vi "auto_irsuccess.vi"(9 "Direction":dbl, 10 "Skip IR":bool) -> (3 "Success":bool)   [LabVIEW 2010, in "LASA Beta.lvrbt"]
uses:
  LASA Beta.lvrbt
  op-run.vi
  op-read.vi
panel:
  # "Output"
  # "Skip IR beacon mode and just place if TRUE"
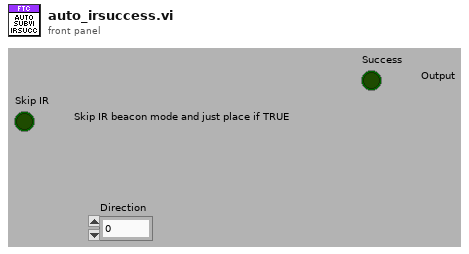
[diagram p1: front panel]
types:
  T1 = enum16{"Initialize", "Drive", "Math", "Move Back", "Exit"}
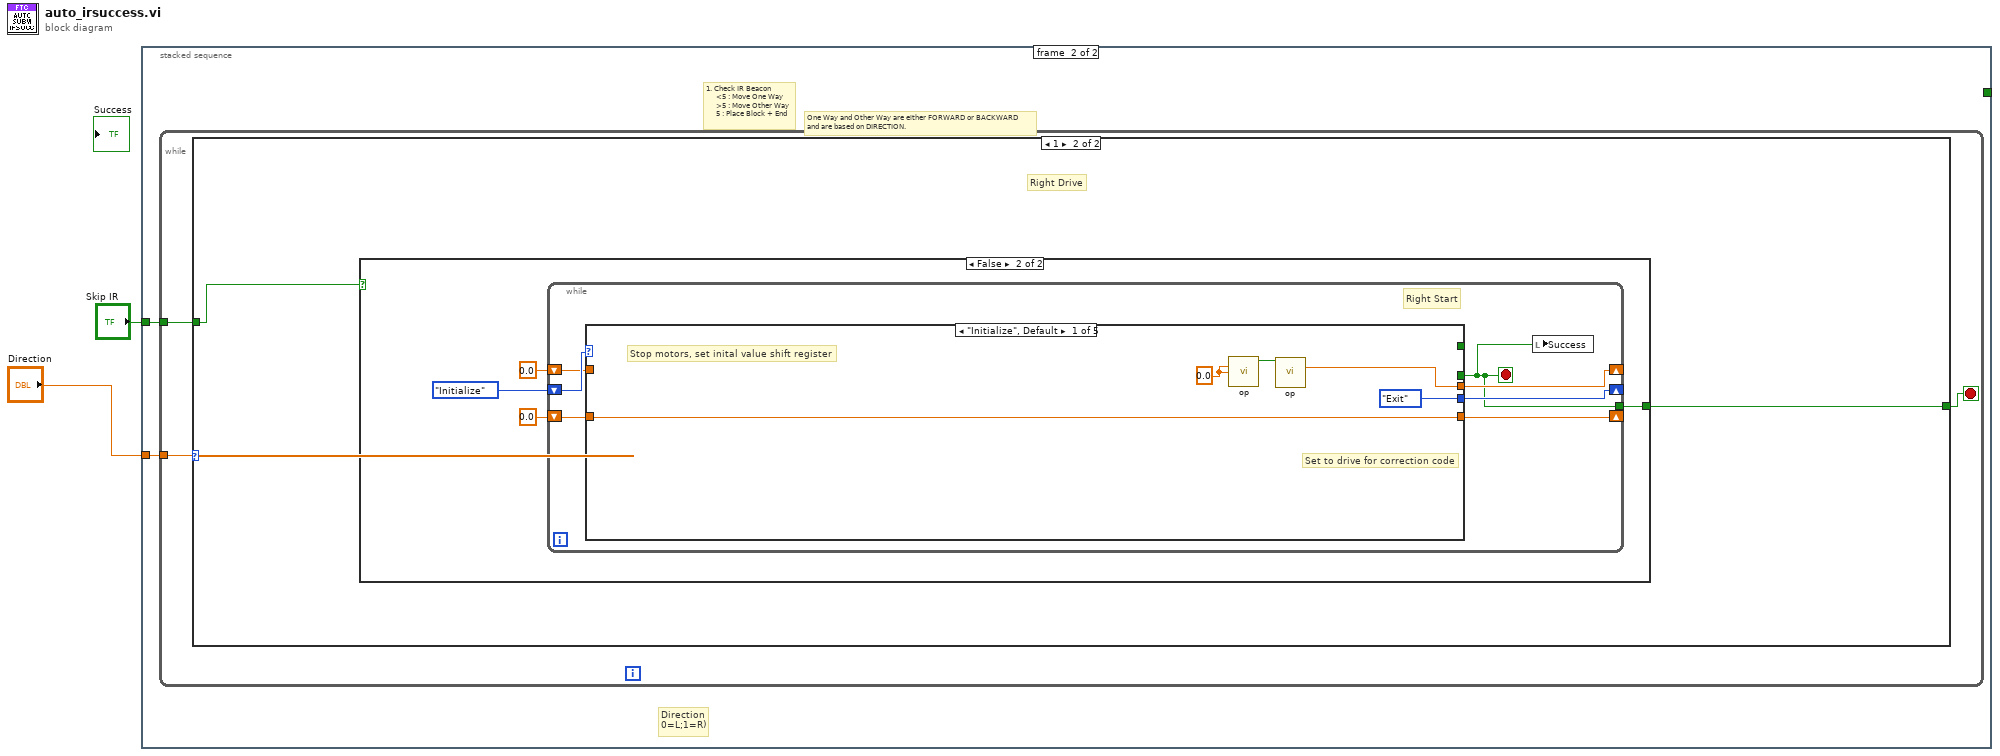
[diagram p0: block diagram]
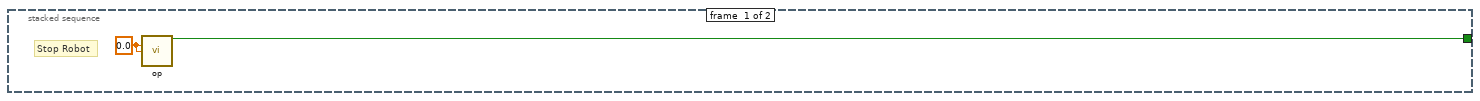
[diagram p2: hidden frame]
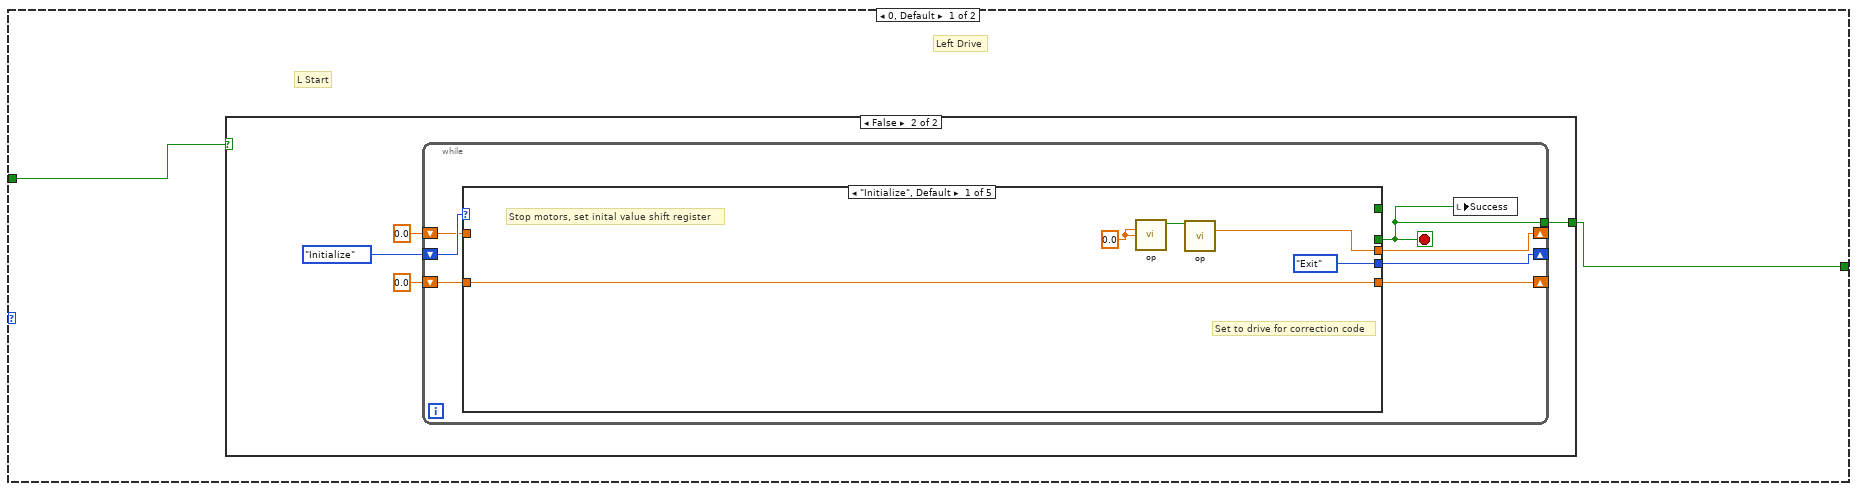
[diagram p3: hidden frame]
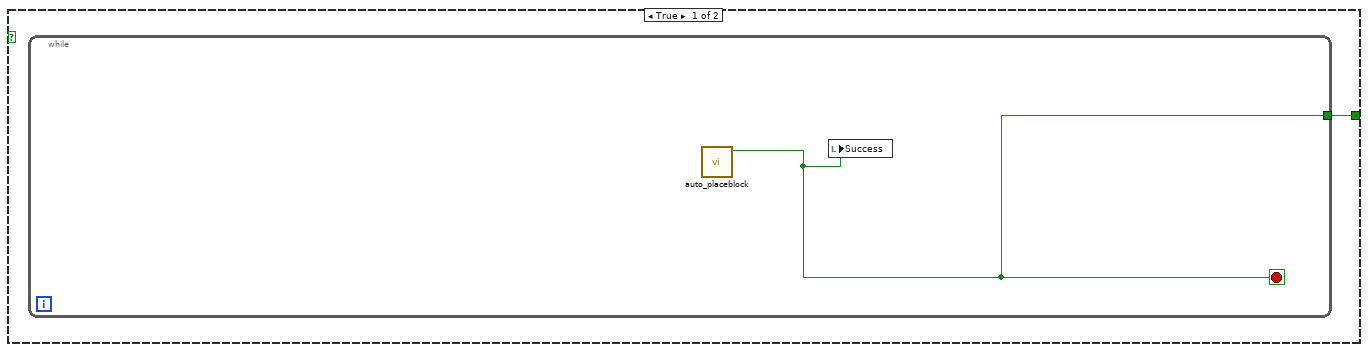
[diagram p4: hidden frame]
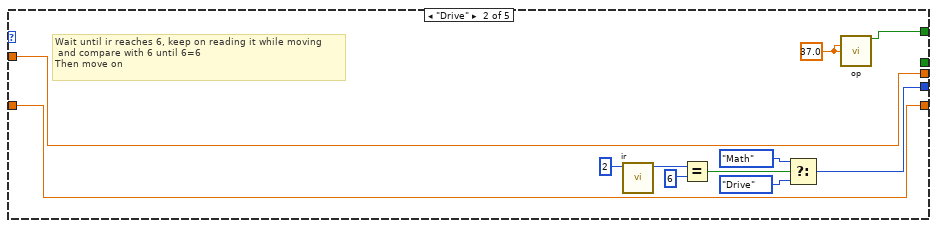
[diagram p5: hidden frame]
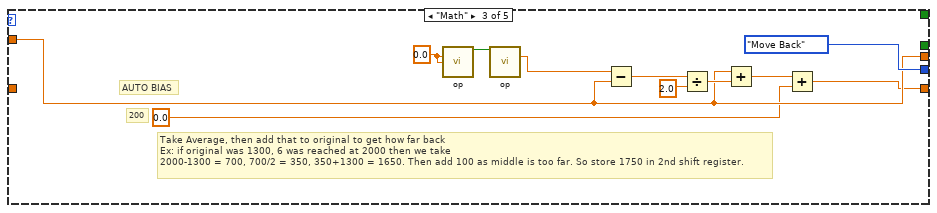
[diagram p6: hidden frame]
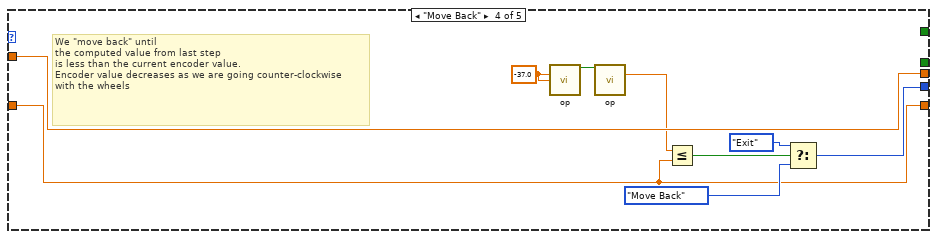
[diagram p7: hidden frame]
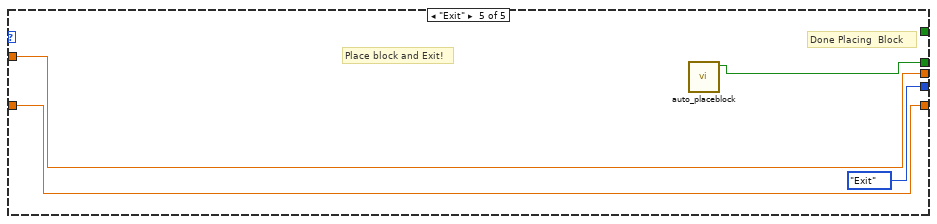
[diagram p8: hidden frame]
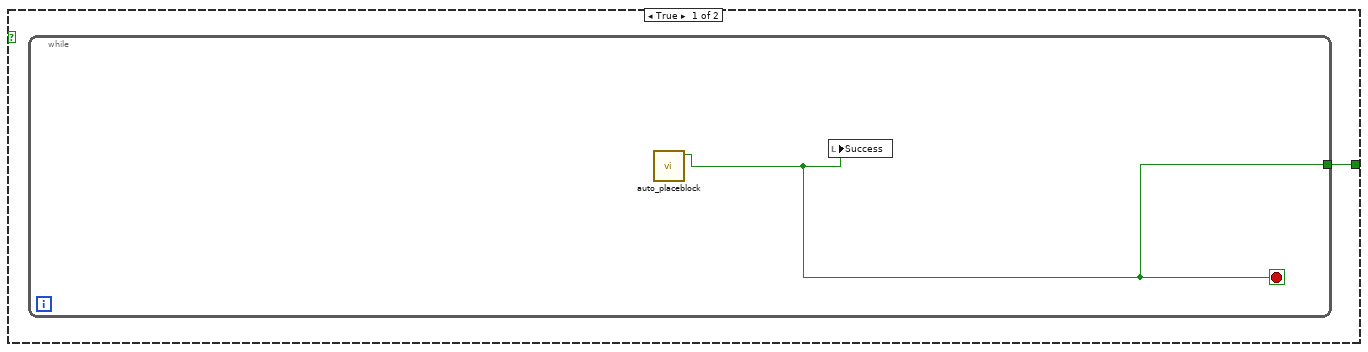
[diagram p9: hidden frame]
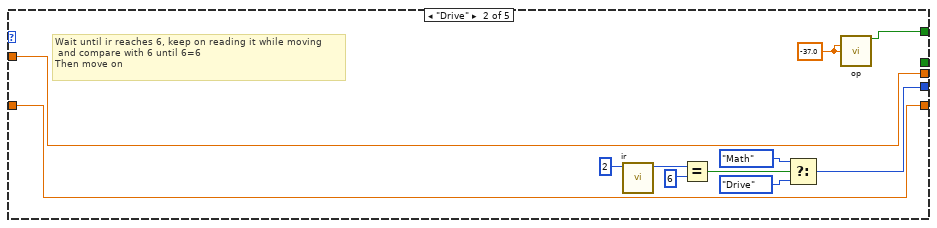
[diagram p10: hidden frame]
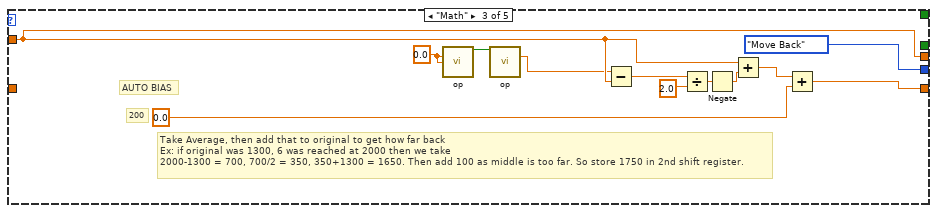
[diagram p11: hidden frame]
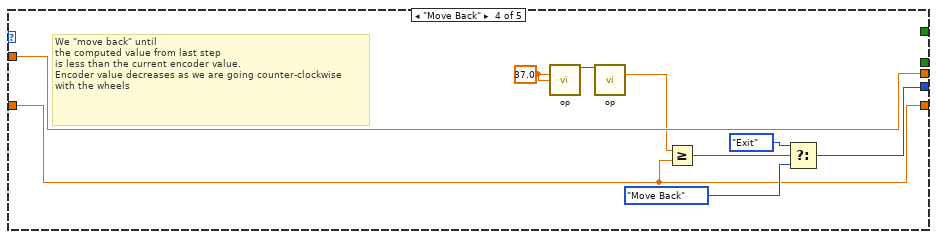
[diagram p12: hidden frame]
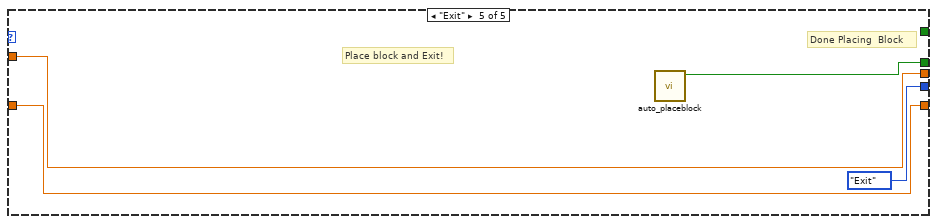
[diagram p13: hidden frame]
diagram:
  n1 = stacked-sequence {
    tunnel: "Skip IR" -> [_ w6]
    tunnel: "Direction" -> [_ w5]
    tunnel: [w3 _] -> _
    frame #0 {
      w4 = 0.0 ("Left Drive")
      # "Stop Robot"
      n2 = call-poly "op.vi"("Left Drive"=w4, "Right Drive"=w4) -> ("Chain OUT"=w3:bool)  [unwired: 13 in]
    }
    frame #1 {
      # "Direction\n0=L;1=R)"
      # "One Way and Other Way are either FORWARD or BACKWARD\nand are based on DIRECTION."
      # "1. Check IR Beacon\n     <5 : Move One Way\n     >5 : Move Other Way\n     5 : Place Block + End"
      n3 = while {
        tunnel: w6 -> [w8]
        tunnel: w5 -> [w9]
        stop <- w7 stop-if-true
        n4 = case shown="1" w9 {
          tunnel: w8 -> [w11 w66]
          tunnel: [w10 w65] -> w7
          frame 0, Default {
            # "Left Drive"
            # "L Start"
            n5 = case shown="False" w11 {
              tunnel: [w12 w14] -> w10
              frame True {
                n6 = while {
                  tunnel: [w13] -> w12
                  stop <- w13 stop-if-true
                  n7 = call "auto_placeblock.vi"() -> ("Chain OUT"=w13:bool)  [unwired: 11 in]
                  n8 = local write "Success"(w13) -> ()
                }
              }
              frame False {
                n9 = while {
                  shift-right: [w23] -> _
                  shift-left: T1."Initialize" -> [w24]
                  shift-right: [w22] -> _
                  shift-left: 0.0 -> [w21]
                  shift-right: [w20] -> _
                  shift-left: 0.0 -> [w19]
                  tunnel: [w18] -> w14
                  stop <- w18 stop-if-true
                  n10 = case shown="\"Initialize\", Default" w24 {
                    tunnel: [T1."Exit" w37 T1."Move Back" w55 T1."Exit"] -> w23
                    tunnel: [w25 w40 w46 w60 w64] -> w22
                    tunnel: w21 -> [_ w40 w46 w60 w64]
                    tunnel: [_ _ _ _ w61] -> w18
                    tunnel: w19 -> [w28 w31 _ w54 w63]
                    tunnel: [w28 w31 w43 w54 w63] -> w20
                    tunnel: [_ w30 _ _ _] -> _
                    frame "Initialize", Default {
                      w27 = 0.0 ("Left Drive")
                      # "Set to drive for correction code"
                      # "Stop motors, set inital value shift register"
                      n11 = call-poly "op.vi"("Left Drive"=w27, "Right Drive"=w27) -> ("Chain OUT"=w26:bool)  [unwired: 13 in]
                      n12 = call-poly "op.vi"("Chain IN"=w26) -> ("Encoder Left Drive"=w25:dbl)  [unwired: 8 in, 6 out]
                    }
                    frame "Drive" {
                      w32 = 37.0 ("Left Drive")
                      # "Wait until ir reaches 6, keep on reading it while moving\n and compare with 6 until 6=6 \nThen move on"
                      n13 = call "ir.vi"("Port"=u8 2) -> ("Direction"=w34:i16)  [unwired: 10 in]
                      n14 = Equal?(x=w34, y=i16 6) -> (x = y?=w33:bool)
                      n15 = Select(t=T1."Math", s=w33, f=T1."Drive") -> (s? t:f=w37:T1)
                      n16 = call-poly "op.vi"("Left Drive"=w32, "Right Drive"=w32) -> ("Chain OUT"=w30:bool)  [unwired: 13 in]
                    }
                    frame "Math" {
                      w51 = 0.0 ("Left Drive")
                      # "AUTO BIAS"
                      # "200"
                      # "Take Average, then add that to original to get how far back\nEx: if original was 1300, 6 was reached at 2000 then we take \n2000-1300 = 700, 700/2 = 350, 350+1300 = 1650. Then add 100 as middle is too far. So store 1750 in 2nd shift register."
                      n17 = call-poly "op.vi"("Left Drive"=w51, "Right Drive"=w51) -> ("Chain OUT"=w42:bool)  [unwired: 13 in]
                      n18 = call-poly "op.vi"("Chain IN"=w42) -> ("Encoder Left Drive"=w41:dbl)  [unwired: 8 in, 6 out]
                      n19 = Subtract(x=w41, y=w46) -> (x-y=w50:dbl)
                      n20 = Divide(x=w50, y=2.0) -> (x/y=w47:dbl)
                      n21 = Add(x=w46, y=w47) -> (x+y=w45:dbl)
                      n22 = Add(x=w45, y=0.0) -> (x+y=w43:dbl)
                    }
                    frame "Move Back" {
                      w57 = -37.0 ("Left Drive")
                      # "We \"move back\" until\nthe computed value from last step\nis less than the current encoder value.\nEncoder value decreases as we are going counter-clockwise\nwith the wheels"
                      n23 = call-poly "op.vi"("Left Drive"=w57, "Right Drive"=w57) -> ("Chain OUT"=w53:bool)  [unwired: 13 in]
                      n24 = call-poly "op.vi"("Chain IN"=w53) -> ("Encoder Left Drive"=w52:dbl)  [unwired: 8 in, 6 out]
                      n25 = Less Or Equal?(x=w52, y=w54) -> (x <= y?=w58:bool)
                      n26 = Select(t=T1."Exit", s=w58, f=T1."Move Back") -> (s? t:f=w55:T1)
                    }
                    frame "Exit" {
                      # "Done Placing  Block"
                      # "Place block and Exit!"
                      n27 = call "auto_placeblock.vi"() -> ("Chain OUT"=w61:bool)  [unwired: 11 in]
                    }
                  }
                  n28 = local write "Success"(w18) -> ()
                }
              }
            }
          }
          frame 1 {
            # "Right Drive"
            # "Right Start"
            n29 = case shown="False" w66 {
              tunnel: [w67 w69] -> w65
              frame True {
                n30 = while {
                  tunnel: [w68] -> w67
                  stop <- w68 stop-if-true
                  n31 = call "auto_placeblock.vi"() -> ("Chain OUT"=w68:bool)  [unwired: 11 in]
                  n32 = local write "Success"(w68) -> ()
                }
              }
              frame False {
                n33 = while {
                  shift-right: [w78] -> _
                  shift-left: T1."Initialize" -> [w79]
                  shift-right: [w77] -> _
                  shift-left: 0.0 -> [w76]
                  shift-right: [w75] -> _
                  shift-left: 0.0 -> [w74]
                  tunnel: [w73] -> w69
                  stop <- w73 stop-if-true
                  n34 = case shown="\"Initialize\", Default" w79 {
                    tunnel: [T1."Exit" w92 T1."Move Back" w111 T1."Exit"] -> w78
                    tunnel: [w80 w95 w102 w116 w120] -> w77
                    tunnel: w76 -> [_ w95 w102 w116 w120]
                    tunnel: [_ _ _ _ w117] -> w73
                    tunnel: w74 -> [w83 w86 _ w110 w119]
                    tunnel: [w83 w86 w99 w110 w119] -> w75
                    tunnel: [_ w85 _ _ _] -> _
                    frame "Initialize", Default {
                      w82 = 0.0 ("Left Drive")
                      # "Set to drive for correction code"
                      # "Stop motors, set inital value shift register"
                      n35 = call-poly "op.vi"("Left Drive"=w82, "Right Drive"=w82) -> ("Chain OUT"=w81:bool)  [unwired: 13 in]
                      n36 = call-poly "op.vi"("Chain IN"=w81) -> ("Encoder Left Drive"=w80:dbl)  [unwired: 8 in, 6 out]
                    }
                    frame "Drive" {
                      w87 = -37.0 ("Left Drive")
                      # "Wait until ir reaches 6, keep on reading it while moving\n and compare with 6 until 6=6 \nThen move on"
                      n37 = call "ir.vi"("Port"=u8 2) -> ("Direction"=w89:i16)  [unwired: 10 in]
                      n38 = Equal?(x=w89, y=i16 6) -> (x = y?=w88:bool)
                      n39 = Select(t=T1."Math", s=w88, f=T1."Drive") -> (s? t:f=w92:T1)
                      n40 = call-poly "op.vi"("Left Drive"=w87, "Right Drive"=w87) -> ("Chain OUT"=w85:bool)  [unwired: 13 in]
                    }
                    frame "Math" {
                      w107 = 0.0 ("Left Drive")
                      # "AUTO BIAS"
                      # "200"
                      # "Take Average, then add that to original to get how far back\nEx: if original was 1300, 6 was reached at 2000 then we take \n2000-1300 = 700, 700/2 = 350, 350+1300 = 1650. Then add 100 as middle is too far. So store 1750 in 2nd shift register."
                      n41 = call-poly "op.vi"("Left Drive"=w107, "Right Drive"=w107) -> ("Chain OUT"=w98:bool)  [unwired: 13 in]
                      n42 = call-poly "op.vi"("Chain IN"=w98) -> ("Encoder Left Drive"=w97:dbl)  [unwired: 8 in, 6 out]
                      n43 = Subtract(x=w97, y=w102) -> (x-y=w106:dbl)
                      n44 = Divide(x=w106, y=2.0) -> (x/y=w103:dbl)
                      n45 = Negate(x=w103) -> (-x=w96:dbl)
                      n46 = Add(x=w102, y=w96) -> (x+y=w101:dbl)
                      n47 = Add(x=w101, y=0.0) -> (x+y=w99:dbl)
                    }
                    frame "Move Back" {
                      w113 = 37.0 ("Left Drive")
                      # "We \"move back\" until\nthe computed value from last step\nis less than the current encoder value.\nEncoder value decreases as we are going counter-clockwise\nwith the wheels"
                      n48 = call-poly "op.vi"("Left Drive"=w113, "Right Drive"=w113) -> ("Chain OUT"=w109:bool)  [unwired: 13 in]
                      n49 = call-poly "op.vi"("Chain IN"=w109) -> ("Encoder Left Drive"=w108:dbl)  [unwired: 8 in, 6 out]
                      n50 = Greater Or Equal?(x=w108, y=w110) -> (x >= y?=w114:bool)
                      n51 = Select(t=T1."Exit", s=w114, f=T1."Move Back") -> (s? t:f=w111:T1)
                    }
                    frame "Exit" {
                      # "Done Placing  Block"
                      # "Place block and Exit!"
                      n52 = call "auto_placeblock.vi"() -> ("Chain OUT"=w117:bool)  [unwired: 11 in]
                    }
                  }
                  n53 = local write "Success"(w73) -> ()
                }
              }
            }
          }
        }
      }
    }
  }
